vi "Generate Dummy Data.vi"(11 "Overroll":i16) -> (0 "Trigger":T1, 3 "Data":i16[](array[numeric]))   [LabVIEW 2014]
uses:
  Trigger Signals.ctl
panel:
  # "Copyright 2014 Vidrio Technologies\nScanImage 5 software is licensed under the Apache License, Version 2.0 (the \"License\"); you may not use any files contained\nwithin the ScanImage 5 release except in compliance with the License. You may obtain a copy of the License at\n http://www.apache.org/licenses/LICENSE-2.0\nUnless required by applicable law or agreed to in writing, software distributed under the License is distributed on an\n\"AS IS\" BASIS, WITHOUT WARRANTIES OR CONDITIONS OF ANY KIND, either express or implied. See the License for the\n specific language governing permissions and limitations under the License."
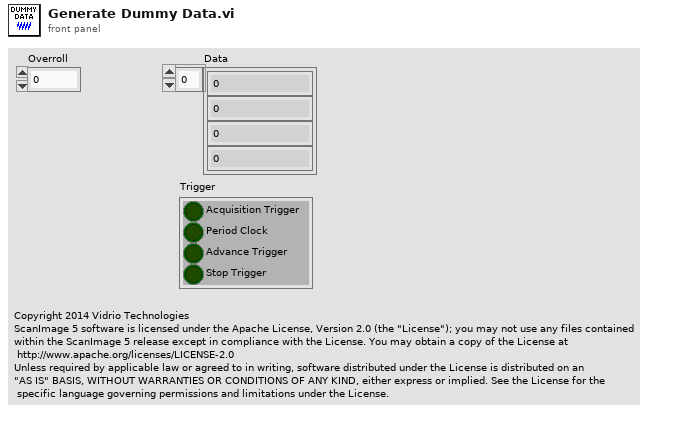
[diagram p1: front panel]
types:
  T1 = typedef "Trigger Signals.ctl" = cluster{"Acquisition Trigger":bool, "Period Clock":bool, "Advance Trigger":bool, "Stop Trigger":bool}
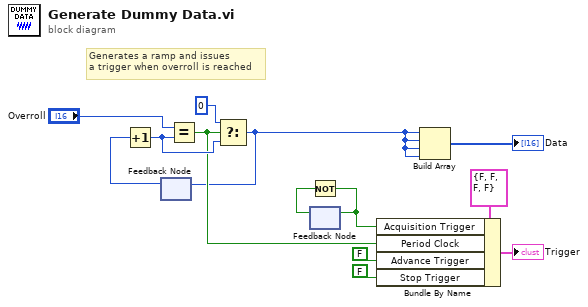
[diagram p0: block diagram]
diagram:
  # "Generates a ramp and issues\na trigger when overroll is reached"
  n1 = feedback #1() -> (w11:i16)  [unwired: 1 in]
  n2 = Increment(x=w11) -> (x+1=w10:i16)
  n3 = Equal?(x="Overroll", y=w10) -> (x = y?=w5:bool)
  n4 = Select(t=i16 0 ("Dummy Start Value"), s=w5, f=w10) -> (s? t:f=w1:i16)
  n5 = feedback-in #1(w1) -> ()
  n6 = feedback #2() -> (w8:bool)  [unwired: 1 in]
  n7 = Not(x=w8) -> (.not. x?=w6:bool)
  n8 = feedback-in #2(w6) -> ()
  n9 = Bundle By Name(cluster=T1 {"Acquisition Trigger"=FALSE, "Period Clock"=FALSE, "Advance Trigger"=FALSE, "Stop Trigger"=FALSE} ("Trigger 2"), "Acquisition Trigger"=w6, "Period Clock"=w5, "Advance Trigger"=FALSE, "Stop Trigger"=FALSE) -> (→"Trigger":T1)
  n10 = Build Array(w1, w1, w1, w1) -> (→"Data":i16[])
